vi "18-Host Requests Equipment Process Program Directory.vi"(8 "error in (no error)":errorcluster) -> (0 "error out":errorcluster, 2 "Timeout?":bool, 3 "PPID":string[](array[string]))   [LabVIEW 2020, in "SECS Scenarios.lvlib" / "Scenarios Class.lvclass"]
uses:
  Scenarios Class.lvclass
  18-Host Requests Equipment Process Program Directory.ctl
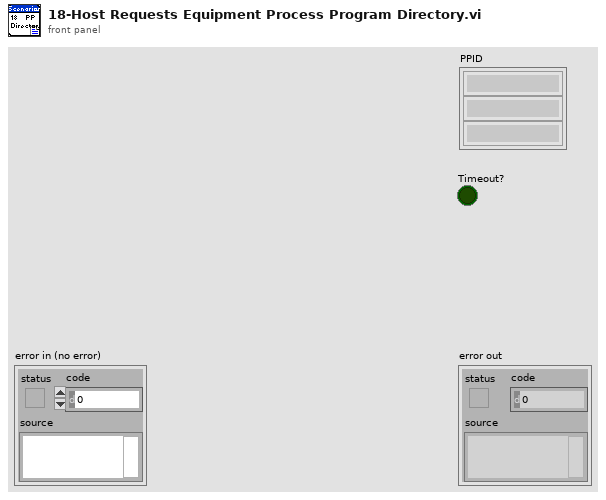
[diagram p1: front panel]
types:
  T1 = typedef "SECS Scenarios.lvlib/Scenarios Class.lvclass/18-Host Requests Equipment Process Program Directory.ctl" = cluster{"Reply Notifier":refnum<notifier>}
  T2 = typedef "SECS Scenarios.lvlib/Scenarios Class.lvclass/Broadcast Refnum.ctl" = cluster{"13-EnableDisable Alarm":refnum<user-event>, "15-Process Program Request":refnum<user-event>, "16-Process Program Send":refnum<user-event>, "17-Deleting a Process Program by Host":refnum<user-event>, "18-Host Requests Equipment Process Program Directory":refnum<user-event>, "19-Equipment Process Program Uploading":refnum<user-event>, "20[1]-Process Program Downloading":refnum<user-event>, "20[2]-Process Program Downloading":refnum<user-event>, "22-Host Sends Information to Equipment":refnum<user-event>, "26-Host Requests to Enter OFF-Line":refnum<user-event>, "27-Host Requests to Enter On-Line":refnum<user-event>, "28[1]-Remote Control[PP-SELECT]":refnum<user-event>, "28[2]-Remote Control[START]":refnum<user-event>, "28[3]-Remote Control[STOP]":refnum<user-event>, "28[4]-Remote Control[LOCAL]":refnum<user-event>, "28[5]-Remote Control[REMOTE]":refnum<user-event>, "28[6]-Remote Control[RCMD]":refnum<user-event>, "30-Host Requests Equipment to Set Time":refnum<user-event>, "31-Host Requests Time Value from Equipment":refnum<user-event>, "32[1]-Trace Data Collection":refnum<user-event>, "32[2]-Trace Data Collection":refnum<user-event>}
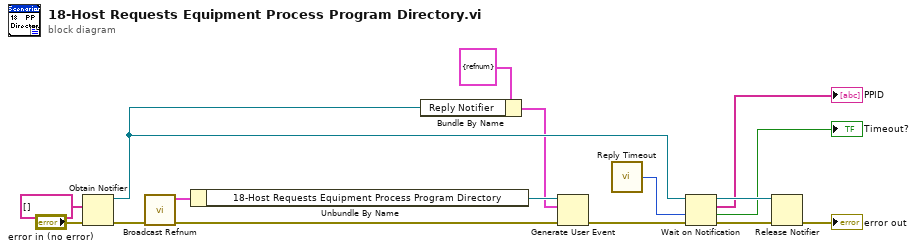
[diagram p0: block diagram]
diagram:
  n1 = Obtain Notifier(notification data type=string[] [], error in (no error)="error in (no error)") -> (notifier out=w3:refnum<notifier>, error out=w15:errorcluster)  [unwired: 2 in, 1 out]
  n2 = call "Broadcast Refnum.vi"("error in"=w15) -> ("error out"=w14:errorcluster, "Broadcast Refnum"=w16:T2)  [unwired: 9 in]
  n3 = Unbundle By Name(w16) -> ("18-Host Requests Equipment Process Program Directory"=w13:refnum<user-event>)
  n4 = Bundle By Name(cluster=T1 {"Reply Notifier"=refnum} ("18-Host Requests Equipment Process Program Directory"), "Reply Notifier"=w3) -> (w2:T1)
  n5 = Generate User Event(user event=w13, event data cluster=w2, error in=w14) -> (error out=w12:errorcluster)  [unwired: 1 in, 1 out]
  n6 = call "Reply Timeout.vi"() -> ("Reply Timeout"=w11:i32)
  n7 = Wait on Notification(notifier=w3, timeout in ms (-1)=w11, error in (no error)=w12) -> (notifier out=w10:refnum<notifier>, notification=→"PPID":string[], timed out?=→"Timeout?":bool, error out=w9:errorcluster)  [unwired: 1 in]
  n8 = Release Notifier(notifier=w10, error in (no error)=w9) -> (error out=→"error out":errorcluster)  [unwired: 1 in, 2 out]
